vi "HTTP Client reqwest Tree.vi"() -> ()   [LabVIEW 2020]
uses:
  <vilib>/VIPM Community/HTTP Client Plugin - Base/Classes/Abstract HTTP Client/Abstract HTTP Client.lvclass
  HTTP Client reqwest.lvclass
  C:/Program Files/National Instruments/LabVIEW 2024/vi.lib/VIPM Community/HTTP Client Plugin - Base/Classes/Abstract HTTP Client/Abstract HTTP Client.lvclass
panel:
  out "Array":string[][](array[string])
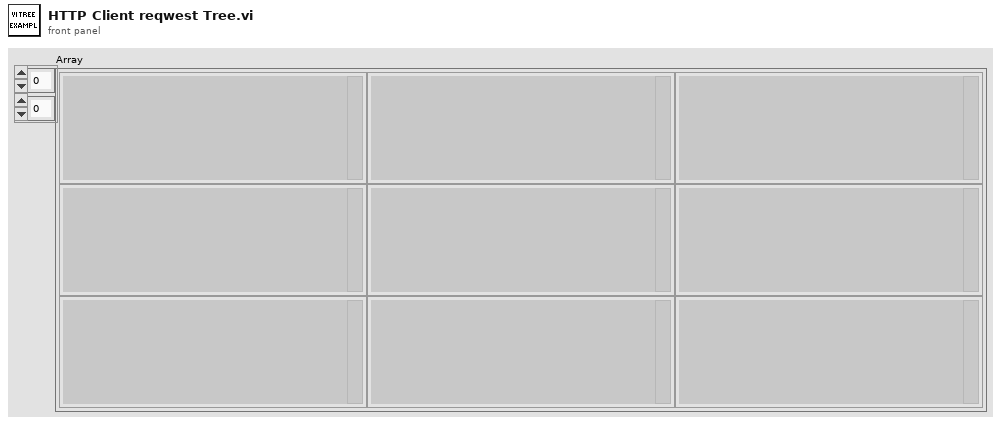
[diagram p1: front panel]
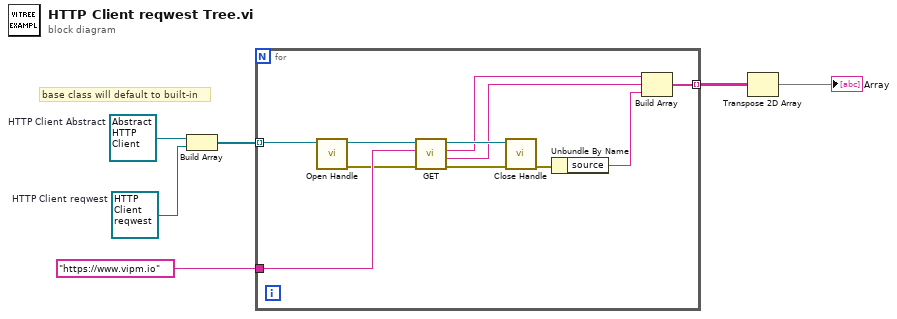
[diagram p0: block diagram]
diagram:
  w1 = refnum<class "HTTP Client reqwest.lvclass"> refnum  # HTTP Client reqwest
  w2 = refnum<class "Abstract HTTP Client.lvclass"> refnum  # HTTP Client Abstract
  # "base class will default to built-in"
  n1 = Build Array(w2, w1) -> (w6:refnum<class "Abstract HTTP Client.lvclass">[])
  n2 = for {
    tunnel: w6 -> [w17] mode=indexing
    tunnel: "https://www.vipm.io" ("url") -> [w14]
    tunnel: [w8] -> w4 mode=indexing
    n3 = call-dynamic "Open Handle.vi"("HTTP Client Abstract in"=w17) -> ("error out"=w13:errorcluster, "HTTP Client Abstract out"=w16:refnum<class "Abstract HTTP Client.lvclass">)  [unwired: 9 in]
    n4 = call-dynamic "GET.vi"("error in (no error)"=w13, "url"=w14, "HTTP Client Abstract in"=w16) -> ("error out"=w12:errorcluster, "body"=w7:string, "headers"=w10:string, "HTTP Client Abstract out"=w15:refnum<class "Abstract HTTP Client.lvclass">)  [unwired: 4 in, 1 out]
    n5 = call-dynamic "Close Handle.vi"("error in (no error)"=w12, "HTTP Client Abstract in"=w15) -> ("error out"=w11:errorcluster)  [unwired: 8 in, 1 out]
    n6 = Unbundle By Name(w11) -> ("source"=w9:string)
    n7 = Build Array(w10, w7, w9) -> (w8:string[])
  }
  n8 = Transpose 2D Array(2D array=w4) -> (transposed array=→"Array":string[][])
